vi "Untitled 3 (SubVI).vi"(9 "Actual Value":dbl, 10 "Percent ceiling":dbl, 11 "Previous set point":dbl) -> (3 "New Set Point":dbl)   [LabVIEW 2012]
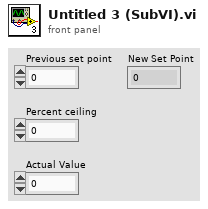
[diagram p1: front panel]
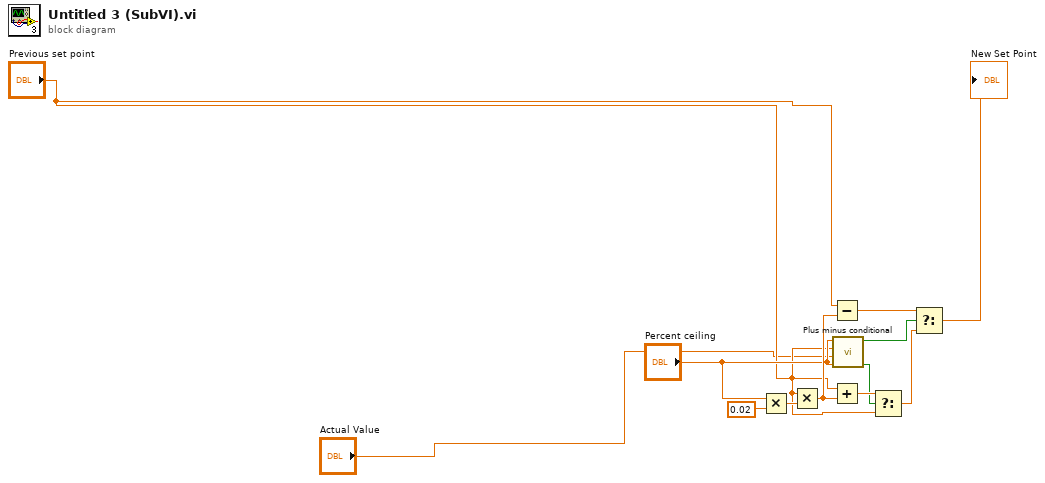
[diagram p0: block diagram]
diagram:
  n1 = Multiply(x="Percent ceiling", y=0.02) -> (x*y=w11:dbl)
  n2 = Multiply(x="Previous set point", y=w11) -> (x*y=w12:dbl)
  n3 = Subtract(x="Previous set point", y=w12) -> (x-y=w6:dbl)
  n4 = Add(x="Previous set point", y=w12) -> (x+y=w7:dbl)
  n5 = call "Plus minus conditional.vi"("Percent Floor"="Percent ceiling", "Actual Number"="Actual Value", "Target"="Previous set point", "Percent ceiling"="Percent ceiling") -> ("Below"=w3:bool, "Above"=w2:bool)  [unwired: 5 in, 1 out]
  n6 = Select(t=w7, s=w3, f="Previous set point") -> (s? t:f=w4:dbl)
  n7 = Select(t=w6, s=w2, f=w4) -> (s? t:f=→"New Set Point":dbl)
